vi "Error_Gen.vi"(6 "Error(T)/Warning":bool=TRUE, 8 "error in":errorcluster, 9 "type of dialog (OK msg:1)":T1=1 items=["no dialog", "OK message", "continue or stop message", "OK message + warnings", "continue/stop + warnings"], 10 "ErrorInfor":variant, 11 "message":string) -> (0 "error out":errorcluster)   [LabVIEW 2015, in "Picture_Class.lvclass"]
uses:
  Picture_Class.lvclass
  <vilib>/Utility/error.llb/DialogType.ctl
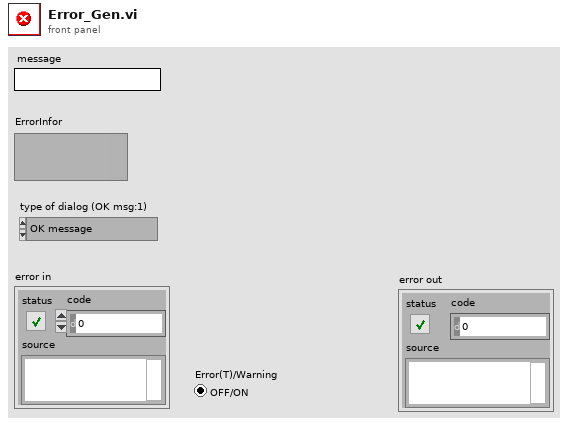
[diagram p1: front panel]
types:
  T1 = typedef "DialogType.ctl" = u16
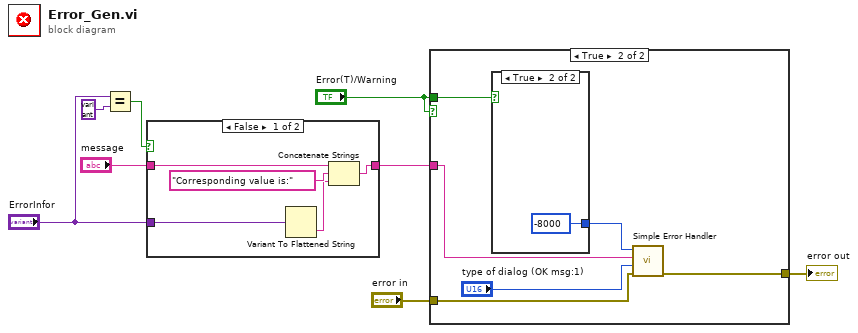
[diagram p0: block diagram]
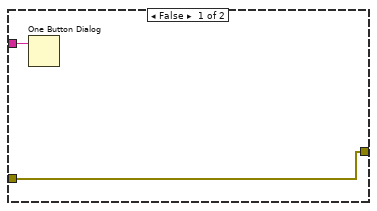
[diagram p2: hidden frame]
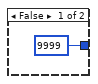
[diagram p3: hidden frame]
diagram:
  n1 = Equal?(x="ErrorInfor", y=variant ("ErrorInfor 2")) -> (x = y?=w7:bool)
  n2 = case shown="False" w7 {
    tunnel: [w12 w14] -> w6
    tunnel: "message" -> [w11 w14]
    tunnel: "ErrorInfor" -> [w10 _]
    frame False {
      n3 = Variant To Flattened String(Variant=w10) -> (data string=w9:string)  [unwired: 1 out]
      n4 = Concatenate Strings(w11, "Corresponding value is:" ("message 2"), w9) -> (w12:string)
    }
    frame True {
    }
  }
  n5 = case shown="True" "Error(T)/Warning" {
    tunnel: "Error(T)/Warning" -> [_ w22]
    tunnel: w6 -> [w15 w20]
    tunnel: "error in" -> [w16 w18]
    tunnel: [w16 w17] -> w1
    frame False {
      n6 = One Button Dialog(message=w15) -> ()  [unwired: 1 in, 1 out]
    }
    frame True {
      n7 = case shown="True" w22 {
        tunnel: [9999 ("code") -8000 ("code")] -> w21
        frame False {
        }
        frame True {
        }
      }
      n8 = call <vilib>:"Simple Error Handler.vi"("error code (no error:0)"=w21, "error source (\" \")"=w20, "type of dialog (OK msg:1)"="type of dialog (OK msg:1)", "error in (no error)"=w18) -> ("error out"=w17:errorcluster)  [unwired: 1 in, 4 out]
    }
  }
  "error out" <- w1
